vi "SafetyStatus.vi"(0 "DashboardServer in":refnum<class "Dashboard Server.lvclass">, 5 "error in (no error)":errorcluster) -> (14 "DashboardServer out":refnum<class "Dashboard Server.lvclass">, 15 "safetyStatus":string, 19 "error out":errorcluster)   [LabVIEW 2019, in "Dashboard Server.lvclass"]
uses:
  Dashboard Server.lvclass
panel:
  out "returnStatus":string
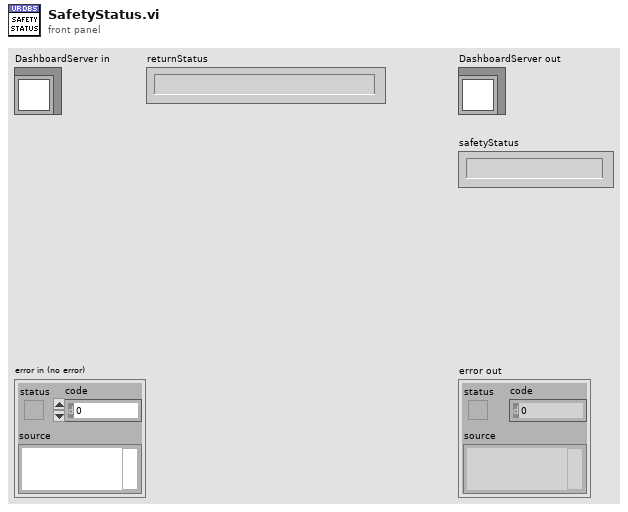
[diagram p1: front panel]
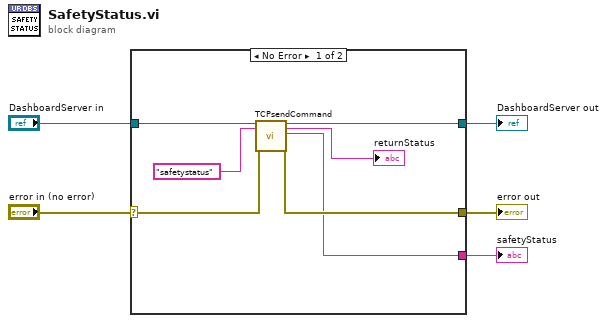
[diagram p0: block diagram]
diagram:
  n1 = case shown="No Error" "error in (no error)" {
    selector: "error in (no error)" -> [w10 w14]
    tunnel: [w9 w14] -> w4
    tunnel: [w11 w13] -> w2
    tunnel: "DashboardServer in" -> [w12 w13]
    tunnel: [w6 _] -> w1
    frame No Error {
      n2 = call "TCPsendCommand.vi"("DashboardServer in"=w12, "command"="safetystatus", "error in (no error)"=w10) -> ("DashboardServer out"=w11:refnum<class "Dashboard Server.lvclass">, "returnStatus"=→"returnStatus":string, "data"=w6:string, "error out"=w9:errorcluster)  [unwired: 13 in]
    }
    frame Error {
    }
  }
  "error out" <- w4
  "DashboardServer out" <- w2
  "safetyStatus" <- w1
